vi "JSON Object Probe.vi"(11 "JSON Object In":refnum<class "JSON Object.lvclass">) -> (2 "Value String":string, 3 "Boolean":bool)   [LabVIEW 2020, in "Library Commun.lvlib" / "JSON Object.lvclass"]
uses:
  JSON Object.lvclass
panel:
  out "JSON":string
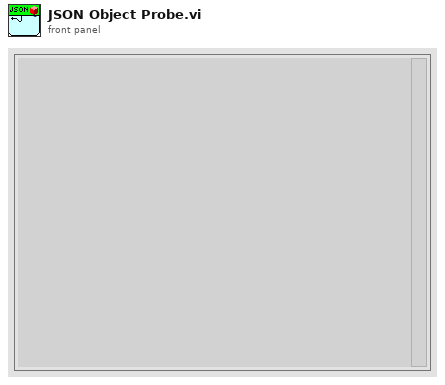
[diagram p1: front panel]
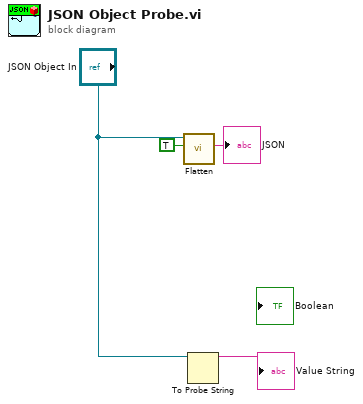
[diagram p0: block diagram]
diagram:
  n1 = call-dynamic "Flatten.vi"("Pretty Print?"=TRUE, "JSON Object in"="JSON Object In") -> ("<JSON>"=→"JSON":string)  [unwired: 8 in, 1 out]
  n2 = To Probe String(7:"JSON Object In") -> (3:→"Value String":string)  [unwired: 2 in, 1 out]
